vi "SubFilter1.vi"(8 "Array1":dbl[](array[numeric]), 9 "N":dbl, 11 "X":dbl) -> (0 "XFiltered":dbl, 3 "Array 2":dbl[](array[numeric]))   [LabVIEW 2011]
uses:
  <vilib>/Analysis/3filter.llb/Filter Passband Type.ctl
  <vilib>/Analysis/3filter.llb/Butterworth Filter (DBL).vi
  <vilib>/Analysis/NI_AALBase.lvlib
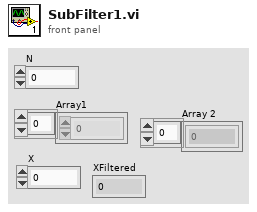
[diagram p1: front panel]
types:
  T1 = typedef "NI_AALBase.lvlib/Filter Passband Type.ctl" = enum32{"Lowpass", "Highpass", "Bandpass", "Bandstop"}
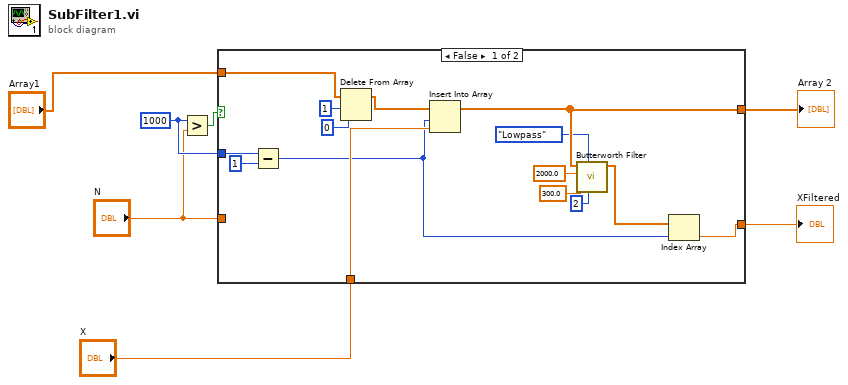
[diagram p0: block diagram]
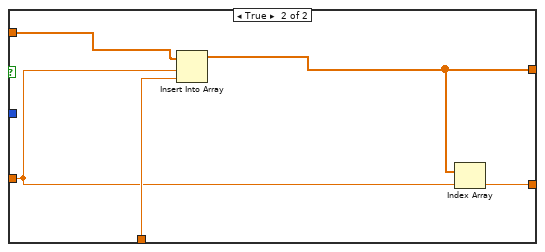
[diagram p2: hidden frame]
diagram:
  w6 = 1000 ("x")
  n1 = Greater?(x=w6, y="N") -> (0:w7:bool)
  n2 = case shown="False" w7 {
    tunnel: "N" -> [_ w25]
    tunnel: w6 -> [w10 _]
    tunnel: "X" -> [w20 w27]
    tunnel: "Array1" -> [w17 w26]
    tunnel: [w16 w24] -> w3
    tunnel: [w9 w23] -> w2
    frame False {
      n3 = Subtract(x=w10, y=1) -> (x-y=w8:i32)
      n4 = Delete From Array(array=w17, length=1, index=0) -> (array with subset deleted=w21:dbl[])  [unwired: 1 out]
      n5 = Insert Into Array(array=w21, index=w8, new element=w20) -> (w16:dbl[])
      n6 = call-poly <vilib>:"Butterworth Filter.vi"("order"=2, "filter type"=Filter_Passband_Type."Lowpass", "low cutoff freq: fl"=300.0, "sampling freq: fs"=2000.0, "X"=w16) -> ("Filtered X"=w11:dbl[])  [unwired: 3 in, 1 out]
      n7 = Index Array(array=w11, index=w8) -> (element=w9:dbl)
    }
    frame True {
      n8 = Insert Into Array(array=w26, index=w25, new element=w27) -> (w24:dbl[])
      n9 = Index Array(array=w24, index=w25) -> (element=w23:dbl)
    }
  }
  "Array 2" <- w3
  "XFiltered" <- w2
